vi "Lock-in Read Sensitivity (SubVI).vi"(8 "error in (no error)":errorcluster, 10 "Voltage measure?":bool, 11 "VISA Refnum in":refnum<visa-resource-name>) -> (0 "error out":errorcluster, 2 "Sensitivity out":dbl, 3 "VISA Refnum out":refnum<visa-resource-name>)   [LabVIEW 2016]
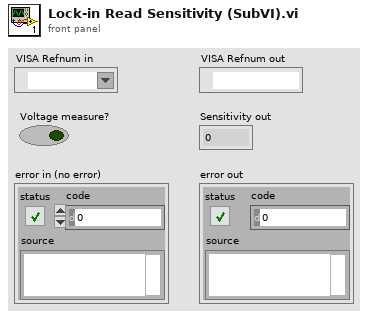
[diagram p1: front panel]
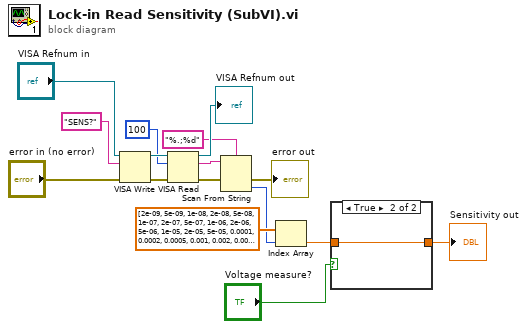
[diagram p0: block diagram]
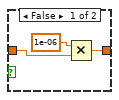
[diagram p2: hidden frame]
diagram:
  n1 = VISA Write(VISA resource name="VISA Refnum in", write buffer="SENS?", error in (no error)="error in (no error)") -> (VISA resource name out=w5:refnum<visa-resource-name>, error out=w2:errorcluster)  [unwired: 1 out]
  n2 = VISA Read(VISA resource name=w5, byte count=u32 100, error in (no error)=w2) -> (VISA resource name out=→"VISA Refnum out":refnum<visa-resource-name>, read buffer=w8:string, error out=w9:errorcluster)  [unwired: 1 out]
  n3 = Scan From String(format string="%.;%d", input string=w8, error in=w9) -> (error out=→"error out":errorcluster, output 1=w7:i32)  [unwired: 2 in, 2 out]
  n4 = Index Array(array=dbl[] [2e-09, 5e-09, 1e-08, 2e-08, 5e-08, 1e-07, 2e-07, 5e-07, 1e-06, 2e-06, 5e-06, 1e-05, 2e-05, 5e-05, 0.0001, 0.0002, 0.0005, 0.001, 0.002, 0.005, 0.01, 0.02, 0.05, 0.1, 0.2, 0.5], index=w7) -> (element=w14:dbl)
  n5 = case shown="True" "Voltage measure?" {
    tunnel: [w17 w20] -> w15
    tunnel: w14 -> [w19 w20]
    frame False {
      n6 = Multiply(x=1e-06, y=w19) -> (x*y=w17:dbl)
    }
    frame True {
    }
  }
  "Sensitivity out" <- w15
